vi "Configure.vi"(8 "error in (no error)":errorcluster, 11 "navX - Interface in":refnum<class "navX - Interface.lvclass">) -> (0 "error out":errorcluster, 3 "navX - Interface out":refnum<class "navX - Interface.lvclass">)   [LabVIEW 2015, in "navX Library v3.lvlib" / "navX - Interface.lvclass"]
uses:
  navX - Interface.lvclass
  navX - Interface.lvclass/navX - Interface.ctl
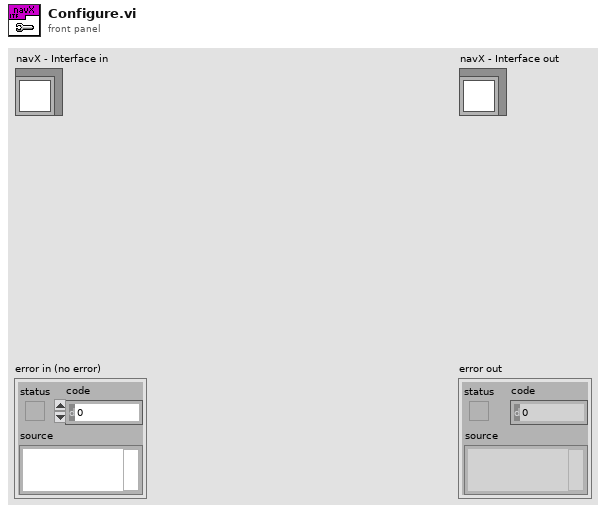
[diagram p1: front panel]
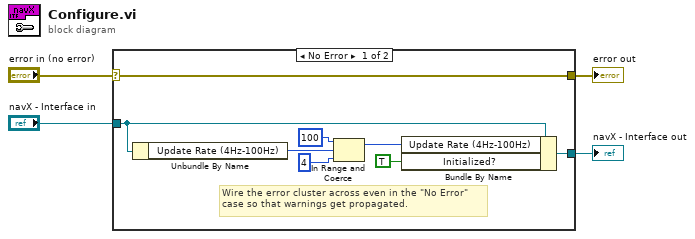
[diagram p0: block diagram]
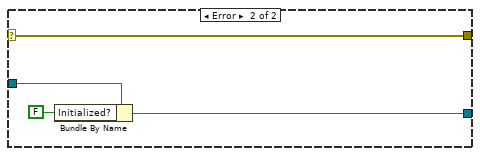
[diagram p2: hidden frame]
diagram:
  n1 = case shown="No Error" "error in (no error)" {
    selector: "error in (no error)" -> [w12 w16]
    tunnel: [w12 w16] -> w3
    tunnel: [w11 w14] -> w1
    tunnel: "navX - Interface in" -> [w10 w15]
    frame No Error {
      # "Wire the error cluster across even in the \"No Error\"\ncase so that warnings get propagated."
      n2 = Unbundle By Name(w10) -> ("Update Rate (4Hz-100Hz)"=w8:u8)
      n3 = In Range and Coerce(upper limit=u8 100, x=w8, lower limit=u8 4) -> (coerced(x)=w7:u8)  [unwired: 1 out]
      n4 = Bundle By Name(cluster=w10, "Update Rate (4Hz-100Hz)"=w7, "Initialized?"=TRUE) -> (w11:refnum<class "navX - Interface.lvclass">)
    }
    frame Error {
      n5 = Bundle By Name(cluster=w15, "Initialized?"=FALSE) -> (w14:refnum<class "navX - Interface.lvclass">)
    }
  }
  "error out" <- w3
  "navX - Interface out" <- w1
